vi "Configure WSS Board.vi"(8 "error in (no error)":errorcluster, 10 "Slot #":T1 max=15, 11 "Rack #":u8) -> (0 "error out":errorcluster, 3 "SPI FIFO Messages":u64[](array[numeric]))   [LabVIEW 2014, in "SLSC configuration Shared.lvlib"]
doc: "Configures the DIO board (IOCON.BANK = 0 - sequential addressing, switch all pins to outputs)."
uses:
  SLSC configuration Shared.lvlib
  SPI Utility/Slot #.ctl
  Constants.vi
  MCP23S17/Update Mode All Pins.vi
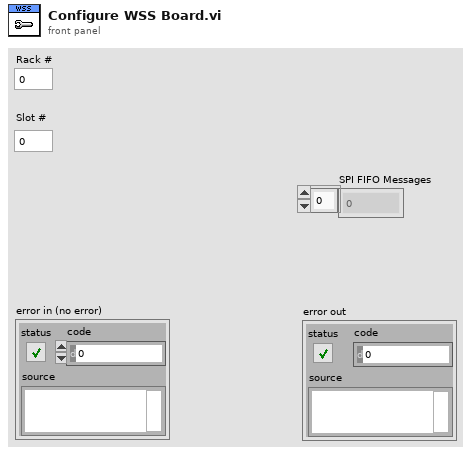
[diagram p1: front panel]
types:
  T1 = typedef "SLSC configuration Shared.lvlib/Slot #.ctl" = u8
  T2 = typedef "SLSC configuration Shared.lvlib/SPI Command.ctl" = cluster{"SPI Command":u32, "Transfer Length":u8}
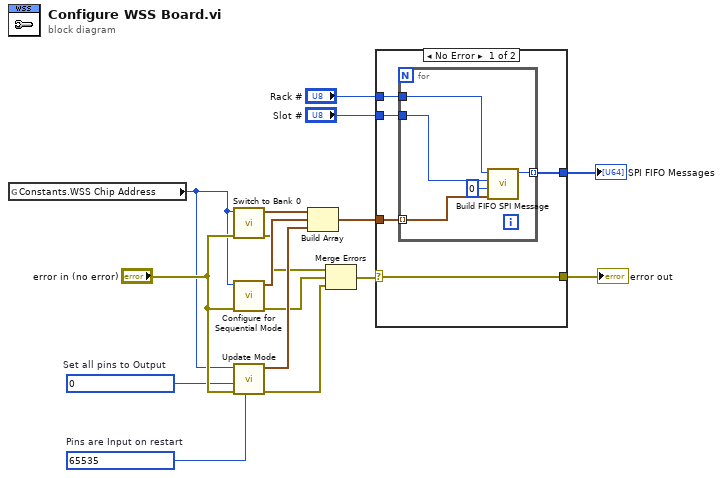
[diagram p0: block diagram]
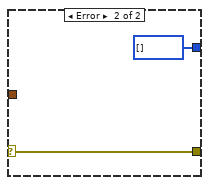
[diagram p2: hidden frame]
diagram:
  w10 = u16 0  # Set all pins to Output
  w11 = u16 65535  # Pins are Input on restart
  n1 = global read "Constants.vi" "Constants.WSS Chip Address"() -> (w12:u8)
  n2 = call "Switch to Bank 0.vi"("error in (no error)"="error in (no error)", "Chip Address (A2 A1 A0)"=w12) -> ("error out"=w5:errorcluster, "SPI Command"=w9:T2)  [unwired: 8 in]
  n3 = call "Configure for Sequential Mode.vi"("error in (no error)"="error in (no error)", "Chip Address (A2 A1 A0)"=w12) -> ("error out"=w4:errorcluster, "SPI Command"=w8:T2)  [unwired: 8 in]
  n4 = call-poly "Update Mode.vi"("Mode Cache in"=w11, "error in (no error)"="error in (no error)", "Mode"=w10, "Chip Address (A2 A1 A0)"=w12) -> ("error out"=w3:errorcluster, "SPI Command"=w7:T2)  [unwired: 5 in, 1 out]
  n5 = Build Array(w9, w8, w7) -> (w6:T2[])
  n6 = Merge Errors(w5, w4, w3) -> (w2:errorcluster)
  n7 = case shown="No Error" w2 {
    selector: w2 -> [w19 w27]
    tunnel: w6 -> [w21 _]
    tunnel: [w20 u64[] []] -> w1
    tunnel: [w19 w27] -> w15
    tunnel: "Slot #" -> [w18 _]
    tunnel: "Rack #" -> [w17 _]
    frame No Error {
      n8 = for {
        tunnel: w21 -> [w25] mode=indexing
        tunnel: [w26] -> w20 mode=indexing
        tunnel: w18 -> [w24]
        tunnel: w17 -> [w23]
        n9 = call "Build FIFO SPI Message.vi"("SPI Command"=w25, "Chip Select"=u8 0, "Slot #"=w24, "Rack #"=w23) -> ("FIFO SPI Message"=w26:u64)  [unwired: 7 in]
      }
    }
    frame Error {
    }
  }
  "SPI FIFO Messages" <- w1
  "error out" <- w15
